vi "App - analyze RUS V6.vi"() -> ()   [LabVIEW 2015] (continued)
"Gamma"=0.06930828334440148, "phase"=3.842055847945363, "Q"=9613.327185902557, "Norm  Ampl"=0.033076114874311065, "z (inf)"=0.3276101846222711-0.3608645481780698i, "4corners"={"z (-pi/2)"=-0.3448645481780698-0.3036101846222711i, "z(inf)"=0.3276101846222711-0.3608645481780698i, "z (pi/2)"=0.3848645481780698+0.3116101846222711i, "z center"=0.020000000000000018+0.0040000000000000036i, "z(0)"=-0.28761018462227106+0.3688645481780698i, "radius"=0.4772317719940016}}, "timestamp(min)"=784.3500000014901, "timestamp"=timestamp(3493774882 s since 1904-01-01), "Magn Field(T)"=0.0}, {"temperature"=82.621, "lorentzian"={"Amplitude"=0.0006972416872469319, "omega(0)"=666.2547956648915, "Gamma"=0.06870985924393977, "phase"=3.8031954056849293, "Q"=9696.6403802327, "Norm  Ampl"=0.0324925976743957, "z (inf)"=0.2945387188362177-0.3771187551409229i, "4corners"={"z (-pi/2)"=-0.3691187551409229-0.2945387188362177i, "z(inf)"=0.2945387188362177-0.3771187551409229i, "z (pi/2)"=0.3771187551409229+0.2865387188362177i, "z center"=0.0040000000000000036-0.0040000000000000036i, "z(0)"=-0.2865387188362177+0.3691187551409229i, "radius"=0.4728957100470491}}, "timestamp(min)"=785.6666666641831, "timestamp"=timestamp(3493774961 s since 1904-01-01), "Magn Field(T)"=0.0}, {"temperature"=82.529, "lorentzian"={"Amplitude"=0.000685912737977901, "omega(0)"=666.2349515696993, "Gamma"=0.06796469782412583, "phase"=3.797698565029673, "Q"=9802.6618656311, "Norm  Ampl"=0.03238343021688376, "z (inf)"=0.29466641947231914-0.3735457173210897i, "4corners"={"z (-pi/2)"=-0.3735457173210897-0.28666641947231913i, "z(inf)"=0.29466641947231914-0.3735457173210897i, "z (pi/2)"=0.3815457173210897+0.29466641947231914i, "z center"=0.0040000000000000036+0.0040000000000000036i, "z(0)"=-0.28666641947231913+0.3815457173210897i, "radius"=0.47647427640571993}}, "timestamp(min)"=787.0, "timestamp"=timestamp(3493775041 s since 1904-01-01), "Magn Field(T)"=0.0}, {"temperature"=82.431, "lorentzian"={"Amplitude"=0.0006963027055650454, "omega(0)"=666.2143601194327, "Gamma"=0.06881606829798663, "phase"=3.7954467351945596, "Q"=9681.087231467485, "Norm  Ampl"=0.03280767739327282, "z (inf)"=0.3019798366954257-0.3744137256418556i, "4corners"={"z (-pi/2)"=-0.3664137256418556-0.2859798366954257i, "z(inf)"=0.3019798366954257-0.3744137256418556i, "z (pi/2)"=0.3904137256418556+0.2939798366954257i, "z center"=0.01200000000000001+0.0040000000000000036i, "z(0)"=-0.2779798366954257+0.3824137256418556i, "radius"=0.47674443200110406}}, "timestamp(min)"=788.3166666701436, "timestamp"=timestamp(3493775120 s since 1904-01-01), "Magn Field(T)"=0.0}, {"temperature"=82.336, "lorentzian"={"Amplitude"=0.0006854343320726252, "omega(0)"=666.1961380017648, "Gamma"=0.06908865385593883, "phase"=3.8305999287252495, "Q"=9642.627274094715, "Norm  Ampl"=0.03292832958384056, "z (inf)"=0.315014801293915-0.3638844014866976i, "4corners"={"z (-pi/2)"=-0.3558844014866976-0.299014801293915i, "z(inf)"=0.315014801293915-0.3638844014866976i, "z (pi/2)"=0.3798844014866976+0.307014801293915i, "z center"=0.01200000000000001+0.0040000000000000036i, "z(0)"=-0.291014801293915+0.3718844014866976i, "radius"=0.4766098012634827}}, "timestamp(min)"=789.6499999985099, "timestamp"=timestamp(3493775200 s since 1904-01-01), "Magn Field(T)"=0.0}, {"temperature"=82.244, "lorentzian"={"Amplitude"=0.0006602362683779066, "omega(0)"=666.1741792701555, "Gamma"=0.0652446126147674, "phase"=3.7900476591164622, "Q"=10210.408991214921, "Norm  Ampl"=0.030878877626074063, "z (inf)"=0.29783931461227364-0.373211480111581i, "4corners"={"z (-pi/2)"=-0.365211480111581-0.28183931461227363i, "z(inf)"=0.29783931461227364-0.373211480111581i, "z (pi/2)"=0.389211480111581+0.28983931461227364i, "z center"=0.01200000000000001+0.0040000000000000036i, "z(0)"=-0.2738393146122736+0.381211480111581i, "radius"=0.4732785802315419}}, "timestamp(min)"=790.9666666686535, "timestamp"=timestamp(3493775279 s since 1904-01-01), "Magn Field(T)"=0.0}, {"temperature"=82.149, "lorentzian"={"Amplitude"=0.0006811288853866493, "omega(0)"=666.1532060539795, "Gamma"=0.06653353924100215, "phase"=3.7827073809377345, "Q"=10012.291750195276, "Norm  Ampl"=0.031598979917904606, "z (inf)"=0.3040523510850292-0.37662541887555895i, "4corners"={"z (-pi/2)"=-0.36062541887555893-0.2800523510850292i, "z(inf)"=0.3040523510850292-0.37662541887555895i, "z (pi/2)"=0.40062541887555897+0.2880523510850292i, "z center"=0.020000000000000018+0.0040000000000000036i, "z(0)"=-0.26405235108502917+0.38462541887555896i, "radius"=0.47493309807922146}}, "timestamp(min)"=792.3000000044703, "timestamp"=timestamp(3493775359 s since 1904-01-01), "Magn Field(T)"=0.0}, {"temperature"=82.054, "lorentzian"={"Amplitude"=0.000661808176586954, "omega(0)"=666.134360050069, "Gamma"=0.06556456826571257, "phase"=3.7898177466936205, "Q"=10159.974780134844, "Norm  Ampl"=0.031199942872906523, "z (inf)"=0.30731473932842324-0.375339694559866i, "4corners"={"z (-pi/2)"=-0.359339694559866-0.2833147393284232i, "z(inf)"=0.30731473932842324-0.375339694559866i, "z (pi/2)"=0.399339694559866+0.2913147393284232i, "z center"=0.020000000000000018+0.0040000000000000036i, "z(0)"=-0.2673147393284232+0.383339694559866i, "radius"=0.475865908953491}}, "timestamp(min)"=793.6166666671634, "timestamp"=timestamp(3493775438 s since 1904-01-01), "Magn Field(T)"=0.0}, {"temperature"=81.963, "lorentzian"={"Amplitude"=0.0007965856787640092, "omega(0)"=666.1144609518154, "Gamma"=0.08199233511572589, "phase"=3.7672280161012996, "Q"=8124.106479119615, "Norm  Ampl"=0.037819800524082445, "z (inf)"=0.2901196948892255-0.3698934585888571i, "4corners"={"z (-pi/2)"=-0.35389345858885707-0.2661196948892255i, "z(inf)"=0.2901196948892255-0.3698934585888571i, "z (pi/2)"=0.3938934585888571+0.2741196948892255i, "z center"=0.020000000000000018+0.0040000000000000036i, "z(0)"=-0.2501196948892255+0.3778934585888571i, "radius"=0.4612601954890381}}, "timestamp(min)"=794.9500000029802, "timestamp"=timestamp(3493775518 s since 1904-01-01), "Magn Field(T)"=0.0}, {"temperature"=81.869, "lorentzian"={"Amplitude"=0.0006443086136346408, "omega(0)"=666.0941688470095, "Gamma"=0.06407247567602045, "phase"=3.7714167781112358, "Q"=10395.948678728824, "Norm  Ampl"=0.030440609010703657, "z (inf)"=0.29183309179237815-0.37994026371105843i, "4corners"={"z (-pi/2)"=-0.3719402637110584-0.27583309179237814i, "z(inf)"=0.29183309179237815-0.37994026371105843i, "z (pi/2)"=0.39594026371105845+0.28383309179237814i, "z center"=0.01200000000000001+0.0040000000000000036i, "z(0)"=-0.26783309179237813+0.38794026371105844i, "radius"=0.4750965011033007}}, "timestamp(min)"=796.2666666656733, "timestamp"=timestamp(3493775597 s since 1904-01-01), "Magn Field(T)"=0.0}, {"temperature"=81.779, "lorentzian"={"Amplitude"=0.0006410550959364764, "omega(0)"=666.0718120080683, "Gamma"=0.06459974834946221, "phase"=3.766353234357599, "Q"=10310.74932993316, "Norm  Ampl"=0.030568951865481662, "z (inf)"=0.2967793225918045-0.37981843110506236i, "4corners"={"z (-pi/2)"=-0.36381843110506235-0.2727793225918045i, "z(inf)"=0.2967793225918045-0.37981843110506236i, "z (pi/2)"=0.4038184311050624+0.2807793225918045i, "z center"=0.020000000000000018+0.0040000000000000036i, "z(0)"=-0.25677932259180447+0.38781843110506237i, "radius"=0.473205432629772}}, "timestamp(min)"=797.6000000014901, "timestamp"=timestamp(3493775677 s since 1904-01-01), "Magn Field(T)"=0.0}, {"temperature"=81.683, "lorentzian"={"Amplitude"=0.0006076266096898992, "omega(0)"=666.0514464195873, "Gamma"=0.06143889388749609, "phase"=3.7181106941402633, "Q"=10840.876263808203, "Norm  Ampl"=0.028912749616661376, "z (inf)"=0.27652437351805453-0.39852955831027087i, "4corners"={"z (-pi/2)"=-0.37452955831027085-0.2605243735180545i, "z(inf)"=0.27652437351805453-0.39852955831027087i, "z (pi/2)"=0.4145295583102709+0.2525243735180545i, "z center"=0.020000000000000018-0.0040000000000000036i, "z(0)"=-0.2365243735180545+0.39052955831027086i, "radius"=0.470593589617759}}, "timestamp(min)"=798.9166666641831, "timestamp"=timestamp(3493775756 s since 1904-01-01), "Magn Field(T)"=0.0}, {"temperature"=81.594, "lorentzian"={"Amplitude"=0.0006072936500237139, "omega(0)"=666.0325514837056, "Gamma"=0.06113714546082676, "phase"=3.728224240712266, "Q"=10894.07342235927, "Norm  Ampl"=0.028993515076990304, "z (inf)"=0.2745182904821208-0.3989495768812215i, "4corners"={"z (-pi/2)"=-0.3829495768812215-0.2665182904821208i, "z(inf)"=0.2745182904821208-0.3989495768812215i, "z (pi/2)"=0.4069495768812215+0.25851829048212077i, "z center"=0.01200000000000001-0.0040000000000000036i, "z(0)"=-0.25051829048212076+0.3909495768812215i, "radius"=0.47423730464432157}}, "timestamp(min)"=800.2333333343267, "timestamp"=timestamp(3493775835 s since 1904-01-01), "Magn Field(T)"=0.0}, {"temperature"=81.501, "lorentzian"={"Amplitude"=0.0005642204027786367, "omega(0)"=666.009795226544, "Gamma"=0.05680859204037456, "phase"=3.653534363936537, "Q"=11723.751131751385, "Norm  Ampl"=0.02670106809576054, "z (inf)"=0.250248223487721-0.4057594372375562i, "4corners"={"z (-pi/2)"=-0.3897594372375562-0.226248223487721i, "z(inf)"=0.250248223487721-0.4057594372375562i, "z (pi/2)"=0.4297594372375562+0.234248223487721i, "z center"=0.020000000000000018+0.0040000000000000036i, "z(0)"=-0.210248223487721+0.4137594372375562i, "radius"=0.4700181281870841}}, "timestamp(min)"=801.5666666701436, "timestamp"=timestamp(3493775915 s since 1904-01-01), "Magn Field(T)"=0.0}, {"temperature"=81.408, "lorentzian"={"Amplitude"=0.0007103334002699531, "omega(0)"=665.9953474434808, "Gamma"=0.07133253713577505, "phase"=3.83036810247925, "Q"=9336.487585964014, "Norm  Ampl"=0.033760580923824425, "z (inf)"=0.3128159431546857-0.36938738782429087i, "4corners"={"z (-pi/2)"=-0.35338738782429086-0.3048159431546857i, "z(inf)"=0.3128159431546857-0.36938738782429087i, "z (pi/2)"=0.3773873878242909+0.2968159431546857i, "z center"=0.01200000000000001-0.0040000000000000036i, "z(0)"=-0.2888159431546857+0.36138738782429086i, "radius"=0.4732844544638054}}, "timestamp(min)"=802.8833333328366, "timestamp"=timestamp(3493775994 s since 1904-01-01), "Magn Field(T)"=0.0}, {"temperature"=81.32, "lorentzian"={"Amplitude"=0.000582609698476251, "omega(0)"=665.9751947106768, "Gamma"=0.05812976574150381, "phase"=3.7119036338106897, "Q"=11456.698409420565, "Norm  Ampl"=0.027685811339377663, "z (inf)"=0.2771384682011788-0.4048972692221223i, "4corners"={"z (-pi/2)"=-0.3808972692221223-0.2611384682011788i, "z(inf)"=0.2771384682011788-0.4048972692221223i, "z (pi/2)"=0.42089726922212234+0.2531384682011788i, "z center"=0.020000000000000018-0.0040000000000000036i, "z(0)"=-0.2371384682011788+0.3968972692221223i, "radius"=0.47627598333172694}}, "timestamp(min)"=804.2000000029802, "timestamp"=timestamp(3493776073 s since 1904-01-01), "Magn Field(T)"=0.0}, {"temperature"=81.229, "lorentzian"={"Amplitude"=0.0006264615993985428, "omega(0)"=665.9553477881376, "Gamma"=0.06192296967531283, "phase"=3.747605050615115, "Q"=10754.57703789096, "Norm  Ampl"=0.02952636058821417, "z (inf)"=0.29959634287061726-0.395914010914744i, "4corners"={"z (-pi/2)"=-0.36391401091474396-0.27559634287061724i, "z(inf)"=0.29959634287061726-0.395914010914744i, "z (pi/2)"=0.419914010914744+0.26759634287061723i, "z center"=0.028000000000000025-0.0040000000000000036i, "z(0)"=-0.2435963428706172+0.387914010914744i, "radius"=0.4768240403041524}}, "timestamp(min)"=805.5333333313465, "timestamp"=timestamp(3493776153 s since 1904-01-01), "Magn Field(T)"=0.0}, {"temperature"=81.134, "lorentzian"={"Amplitude"=0.0005982305706101968, "omega(0)"=665.9343195300057, "Gamma"=0.060064378770215206, "phase"=3.6726072791552684, "Q"=11087.009191881129, "Norm  Ampl"=0.028368216383599845, "z (inf)"=0.25917513837394046-0.41125859074294846i, "4corners"={"z (-pi/2)"=-0.38725859074294844-0.24317513837394047i, "z(inf)"=0.25917513837394046-0.41125859074294846i, "z (pi/2)"=0.4272585907429485+0.23517513837394047i, "z center"=0.020000000000000018-0.0040000000000000036i, "z(0)"=-0.21917513837394045+0.40325859074294845i, "radius"=0.4722968415627252}}, "timestamp(min)"=806.8500000014901, "timestamp"=timestamp(3493776232 s since 1904-01-01), "Magn Field(T)"=0.0}, {"temperature"=81.047, "lorentzian"={"Amplitude"=0.0005436604150965886, "omega(0)"=665.9126957276022, "Gamma"=0.054391615502220096, "phase"=3.623436848836922, "Q"=12242.929164338238, "Norm  Ampl"=0.025547222809101933, "z (inf)"=0.23766121910248528-0.4122123499501512i, "4corners"={"z (-pi/2)"=-0.3962123499501512-0.21366121910248526i, "z(inf)"=0.23766121910248528-0.4122123499501512i, "z (pi/2)"=0.43621234995015123+0.22166121910248526i, "z center"=0.020000000000000018+0.0040000000000000036i, "z(0)"=-0.19766121910248524+0.4202123499501512i, "radius"=0.4696904582298934}}, "timestamp(min)"=808.183333337307, "timestamp"=timestamp(3493776312 s since 1904-01-01), "Magn Field(T)"=0.0}, {"temperature"=80.958, "lorentzian"={"Amplitude"=0.0005359009844102671, "omega(0)"=665.893856538965, "Gamma"=0.05365668737469352, "phase"=3.6524069233354184, "Q"=12410.267743308827, "Norm  Ampl"=0.025203485884419292, "z (inf)"=0.24163913197447767-0.405756529475521i, "4corners"={"z (-pi/2)"=-0.397756529475521-0.22563913197447766i, "z(inf)"=0.24163913197447767-0.405756529475521i, "z (pi/2)"=0.421756529475521+0.23363913197447767i, "z center"=0.01200000000000001+0.0040000000000000036i, "z(0)"=-0.21763913197447765+0.413756529475521i, "radius"=0.46971751551524565}}, "timestamp(min)"=809.5, "timestamp"=timestamp(3493776391 s since 1904-01-01), "Magn Field(T)"=0.0}, {"temperature"=80.871, "lorentzian"={"Amplitude"=0.0005271309388079498, "omega(0)"=665.8735587517352, "Gamma"=0.0529251400813889, "phase"=3.6114149158792337, "Q"=12581.422698697577, "Norm  Ampl"=0.025135729535680076, "z (inf)"=0.23501395823116833-0.41947062787261763i, "4corners"={"z (-pi/2)"=-0.4034706278726176-0.2110139582311683i, "z(inf)"=0.23501395823116833-0.41947062787261763i, "z (pi/2)"=0.44347062787261765+0.21901395823116832i, "z center"=0.020000000000000018+0.0040000000000000036i, "z(0)"=-0.1950139582311683+0.42747062787261764i, "radius"=0.47492986314303676}}, "timestamp(min)"=810.8166666701436, "timestamp"=timestamp(3493776470 s since 1904-01-01), "Magn Field(T)"=0.0}, {"temperature"=80.778, "lorentzian"={"Amplitude"=0.0005267654786186403, "omega(0)"=665.8525097864081, "Gamma"=0.052338348231804756, "phase"=3.5786985819989203, "Q"=12722.077258483016, "Norm  Ampl"=0.024789112532138686, "z (inf)"=0.22049751946201726-0.4331013206689819i, "4corners"={"z (-pi/2)"=-0.40910132066898186-0.20449751946201725i, "z(inf)"=0.22049751946201726-0.4331013206689819i, "z (pi/2)"=0.4491013206689819+0.19649751946201724i, "z center"=0.020000000000000018-0.0040000000000000036i, "z(0)"=-0.18049751946201723+0.4251013206689819i, "radius"=0.47363192323816855}}, "timestamp(min)"=812.1499999985099, "timestamp"=timestamp(3493776550 s since 1904-01-01), "Magn Field(T)"=0.0}, {"temperature"=80.688, "lorentzian"={"Amplitude"=0.0005087274085603998, "omega(0)"=665.8348091435408, "Gamma"=0.05138178107814259, "phase"=3.594454792183561, "Q"=12958.577829969032, "Norm  Ampl"=0.024069545346628345, "z (inf)"=0.22496393075941817-0.42522515487487184i, "4corners"={"z (-pi/2)"=-0.4012251548748718-0.20896393075941816i, "z(inf)"=0.22496393075941817-0.42522515487487184i, "z (pi/2)"=0.44122515487487185+0.20096393075941815i, "z center"=0.020000000000000018-0.0040000000000000036i, "z(0)"=-0.18496393075941814+0.41722515487487183i, "radius"=0.46844513447330344}}, "timestamp(min)"=813.4666666686535, "timestamp"=timestamp(3493776629 s since 1904-01-01), "Magn Field(T)"=0.0}, {"temperature"=80.602, "lorentzian"={"Amplitude"=0.0004882899356981653, "omega(0)"=665.8124994707074, "Gamma"=0.04910380713640485, "phase"=3.547437034982565, "Q"=13559.284672594838, "Norm  Ampl"=0.023246840914470077, "z (inf)"=0.20690464043593387-0.4389659744864196i, "4corners"={"z (-pi/2)"=-0.4149659744864196-0.19090464043593386i, "z(inf)"=0.20690464043593387-0.4389659744864196i, "z (pi/2)"=0.4549659744864196+0.18290464043593385i, "z center"=0.020000000000000018-0.0040000000000000036i, "z(0)"=-0.16690464043593384+0.4309659744864196i, "radius"=0.4734223733384454}}, "timestamp(min)"=814.8000000044703, "timestamp"=timestamp(3493776709 s since 1904-01-01), "Magn Field(T)"=0.0}, {"temperature"=80.512, "lorentzian"={"Amplitude"=0.0004667929339879065, "omega(0)"=665.7921823307441, "Gamma"=0.046744260040372576, "phase"=3.511637879553154, "Q"=14243.292796927488, "Norm  Ampl"=0.022223516509620588, "z (inf)"=0.19194204316769328-0.4472464791600908i, "4corners"={"z (-pi/2)"=-0.4232464791600908-0.17594204316769327i, "z(inf)"=0.19194204316769328-0.4472464791600908i, "z (pi/2)"=0.4632464791600908+0.16794204316769326i, "z center"=0.020000000000000018-0.0040000000000000036i, "z(0)"=-0.15194204316769325+0.4392464791600908i, "radius"=0.4754277100637885}}, "timestamp(min)"=816.1166666671634, "timestamp"=timestamp(3493776788 s since 1904-01-01), "Magn Field(T)"=0.0}, {"temperature"=80.428, "lorentzian"={"Amplitude"=0.0004489209270346126, "omega(0)"=665.770336097026, "Gamma"=0.044967586490377534, "phase"=3.4772880687633405, "Q"=14805.560806326395, "Norm  Ampl"=0.021387258385219494, "z (inf)"=0.1766798725688283-0.45306685491684434i, "4corners"={"z (-pi/2)"=-0.4290668549168443-0.1606798725688283i, "z(inf)"=0.1766798725688283-0.45306685491684434i, "z (pi/2)"=0.46906685491684436+0.15267987256882828i, "z center"=0.020000000000000018-0.0040000000000000036i, "z(0)"=-0.13667987256882827+0.44506685491684433i, "radius"=0.475614994142416}}, "timestamp(min)"=817.433333337307, "timestamp"=timestamp(3493776867 s since 1904-01-01), "Magn Field(T)"=0.0}, {"temperature"=80.338, "lorentzian"={"Amplitude"=0.00044807774453631103, "omega(0)"=665.751169981811, "Gamma"=0.044783012994154305, "phase"=3.478549048664672, "Q"=14866.154049722247, "Norm  Ampl"=0.021488852823685116, "z (inf)"=0.17864413626604192-0.45685996368629533i, "4corners"={"z (-pi/2)"=-0.4328599636862953-0.1626441362660419i, "z(inf)"=0.17864413626604192-0.45685996368629533i, "z (pi/2)"=0.47285996368629535+0.1546441362660419i, "z center"=0.020000000000000018-0.0040000000000000036i, "z(0)"=-0.13864413626604188+0.4488599636862953i, "radius"=0.4798438378072091}}, "timestamp(min)"=818.7666666656733, "timestamp"=timestamp(3493776947 s since 1904-01-01), "Magn Field(T)"=0.0}, {"temperature"=80.249, "lorentzian"={"Amplitude"=0.0004339429327407474, "omega(0)"=665.7310500779857, "Gamma"=0.042797667772295565, "phase"=3.467881219083677, "Q"=15555.311416033208, "Norm  Ampl"=0.02057222058744532, "z (inf)"=0.17407396257240368-0.45932385686764793i, "4corners"={"z (-pi/2)"=-0.4353238568676479-0.15807396257240366i, "z(inf)"=0.17407396257240368-0.45932385686764793i, "z (pi/2)"=0.47532385686764794+0.15007396257240366i, "z center"=0.020000000000000018-0.0040000000000000036i, "z(0)"=-0.13407396257240364+0.4513238568676479i, "radius"=0.48068555270113206}}, "timestamp(min)"=820.0833333358169, "timestamp"=timestamp(3493777026 s since 1904-01-01), "Magn Field(T)"=0.0}, {"temperature"=80.163, "lorentzian"={"Amplitude"=0.0004318053404680994, "omega(0)"=665.7095388817693, "Gamma"=0.04251465906133632, "phase"=3.4410157944541444, "Q"=15658.352991172846, "Norm  Ampl"=0.020516700930109627, "z (inf)"=0.1623460091556352-0.4651079510202824i, "4corners"={"z (-pi/2)"=-0.4411079510202824-0.1463460091556352i, "z(inf)"=0.1623460091556352-0.4651079510202824i, "z (pi/2)"=0.4811079510202824+0.1383460091556352i, "z center"=0.020000000000000018-0.0040000000000000036i, "z(0)"=-0.12234600915563518+0.4571079510202824i, "radius"=0.4825794533718353}}, "timestamp(min)"=821.3999999985099, "timestamp"=timestamp(3493777105 s since 1904-01-01), "Magn Field(T)"=0.0}, {"temperature"=80.075, "lorentzian"={"Amplitude"=0.0004410954482919087, "omega(0)"=665.6890167901994, "Gamma"=0.043283815856253634, "phase"=3.455890711993292, "Q"=15379.628704663312, "Norm  Ampl"=0.021014667550651542, "z (inf)"=0.16209451338682376-0.46572534970148993i, "4corners"={"z (-pi/2)"=-0.4497253497014899-0.15409451338682376i, "z(inf)"=0.16209451338682376-0.46572534970148993i, "z (pi/2)"=0.47372534970148994+0.14609451338682375i, "z center"=0.01200000000000001-0.0040000000000000036i, "z(0)"=-0.13809451338682374+0.4577253497014899i, "radius"=0.4855086626475274}}, "timestamp(min)"=822.7333333343267, "timestamp"=timestamp(3493777185 s since 1904-01-01), "Magn Field(T)"=0.0}, {"temperature"=79.991, "lorentzian"={"Amplitude"=0.00045081873601942116, "omega(0)"=665.666392459161, "Gamma"=0.04417730101978429, "phase"=3.41518632314404, "Q"=15068.06384937482, "Norm  Ampl"=0.021340141879038124, "z (inf)"=0.1425186302592478-0.46908996594687835i, "4corners"={"z (-pi/2)"=-0.45308996594687834-0.1345186302592478i, "z(inf)"=0.1425186302592478-0.46908996594687835i, "z (pi/2)"=0.47708996594687836+0.12651863025924778i, "z center"=0.01200000000000001-0.0040000000000000036i, "z(0)"=-0.11851863025924778+0.46108996594687834i, "radius"=0.48305671434027153}}, "timestamp(min)"=824.0500000044703, "timestamp"=timestamp(3493777264 s since 1904-01-01), "Magn Field(T)"=0.0}, {"temperature"=79.903, "lorentzian"={"Amplitude"=0.00041982693484479076, "omega(0)"=665.6483705534005, "Gamma"=0.04131522725547794, "phase"=3.4489219493632968, "Q"=16111.453688425323, "Norm  Ampl"=0.019830531774632107, "z (inf)"=0.15720110058856143-0.461491616562412i, "4corners"={"z (-pi/2)"=-0.445491616562412-0.14920110058856142i, "z(inf)"=0.15720110058856143-0.461491616562412i, "z (pi/2)"=0.469491616562412+0.14120110058856142i, "z center"=0.01200000000000001-0.0040000000000000036i, "z(0)"=-0.1332011005885614+0.453491616562412i, "radius"=0.4799811859198426}}, "timestamp(min)"=825.3833333328366, "timestamp"=timestamp(3493777344 s since 1904-01-01), "Magn Field(T)"=0.0}, {"temperature"=79.817, "lorentzian"={"Amplitude"=0.0004473207739177375, "omega(0)"=665.6281709996543, "Gamma"=0.04424370195385826, "phase"=3.458741913142453, "Q"=15044.585819103422, "Norm  Ampl"=0.021108986152116926, "z (inf)"=0.1607902810627609-0.4573130004493936i, "4corners"={"z (-pi/2)"=-0.4413130004493936-0.15279028106276088i, "z(inf)"=0.1607902810627609-0.4573130004493936i, "z (pi/2)"=0.4653130004493936+0.14479028106276087i, "z center"=0.01200000000000001-0.0040000000000000036i, "z(0)"=-0.13679028106276087+0.4493130004493936i, "radius"=0.47710714112782604}}, "timestamp(min)"=826.7000000029802, "timestamp"=timestamp(3493777423 s since 1904-01-01), "Magn Field(T)"=0.0}, {"temperature"=79.734, "lorentzian"={"Amplitude"=0.0004310190190592046, "omega(0)"=665.6073287703097, "Gamma"=0.04260556553164946, "phase"=3.3897140798024243, "Q"=15622.544155079097, "Norm  Ampl"=0.020208251339171045, "z (inf)"=0.13648267088154692-0.46378460946108147i, "4corners"={"z (-pi/2)"=-0.43978460946108144-0.12048267088154692i, "z(inf)"=0.13648267088154692-0.46378460946108147i, "z (pi/2)"=0.4797846094610815+0.11248267088154691i, "z center"=0.020000000000000018-0.0040000000000000036i, "z(0)"=-0.0964826708815469+0.45578460946108146i, "radius"=0.47431013030819613}}, "timestamp(min)"=828.0166666656733, "timestamp"=timestamp(3493777502 s since 1904-01-01), "Magn Field(T)"=0.0}, {"temperature"=79.645, "lorentzian"={"Amplitude"=0.0004937499674397325, "omega(0)"=665.5905919172243, "Gamma"=0.04842744547368939, "phase"=3.596201043814433, "Q"=13744.078082310563, "Norm  Ampl"=0.02365453214362621, "z (inf)"=0.2264848572256194-0.43484234277978495i, "4corners"={"z (-pi/2)"=-0.42684234277978494-0.21048485722561938i, "z(inf)"=0.2264848572256194-0.43484234277978495i, "z (pi/2)"=0.45084234277978497+0.2184848572256194i, "z center"=0.01200000000000001+0.0040000000000000036i, "z(0)"=-0.20248485722561937+0.44284234277978496i, "radius"=0.48845302312048866}}, "timestamp(min)"=829.3500000014901, "timestamp"=timestamp(3493777582 s since 1904-01-01), "Magn Field(T)"=0.0}, {"temperature"=79.564, "lorentzian"={"Amplitude"=0.00040885006198574856, "omega(0)"=665.5700736081353, "Gamma"=0.04004258239584053, "phase"=3.476858345479039, "Q"=16621.557197002167, "Norm  Ampl"=0.019088365277797854, "z (inf)"=0.17684441669665446-0.4541603007110035i, "4corners"={"z (-pi/2)"=-0.4301603007110035-0.16084441669665445i, "z(inf)"=0.17684441669665446-0.4541603007110035i, "z (pi/2)"=0.4701603007110035+0.15284441669665444i, "z center"=0.020000000000000018-0.0040000000000000036i, "z(0)"=-0.13684441669665443+0.4461603007110035i, "radius"=0.47670165448122254}}, "timestamp(min)"=830.6666666641831, "timestamp"=timestamp(3493777661 s since 1904-01-01), "Magn Field(T)"=0.0}, {"temperature"=79.476, "lorentzian"={"Amplitude"=0.00042495979141987184, "omega(0)"=665.5494957126687, "Gamma"=0.04195737945665875, "phase"=3.493368033553565, "Q"=15862.51344415277, "Norm  Ampl"=0.01992681463808725, "z (inf)"=0.1836442305829716-0.44984637431067337i, "4corners"={"z (-pi/2)"=-0.42584637431067335-0.1676442305829716i, "z(inf)"=0.1836442305829716-0.44984637431067337i, "z (pi/2)"=0.4658463743106734+0.15964423058297159i, "z center"=0.020000000000000018-0.0040000000000000036i, "z(0)"=-0.14364423058297157+0.44184637431067336i, "radius"=0.4749299145021988}}, "timestamp(min)"=831.9833333343267, "timestamp"=timestamp(3493777740 s since 1904-01-01), "Magn Field(T)"=0.0}, {"temperature"=79.39, "lorentzian"={"Amplitude"=0.00038786955968295433, "omega(0)"=665.5288680893714, "Gamma"=0.03759056507164493, "phase"=3.4134184071386273, "Q"=17704.678469741568, "Norm  Ampl"=0.01789292667738704, "z (inf)"=0.1478002232066598-0.46251770545494364i, "4corners"={"z (-pi/2)"=-0.4385177054549436-0.1318002232066598i, "z(inf)"=0.1478002232066598-0.46251770545494364i, "z (pi/2)"=0.47851770545494365+0.12380022320665979i, "z center"=0.020000000000000018-0.0040000000000000036i, "z(0)"=-0.10780022320665977+0.45451770545494363i, "radius"=0.475995150466198}}, "timestamp(min)"=833.3166666701436, "timestamp"=timestamp(3493777820 s since 1904-01-01), "Magn Field(T)"=0.0}, {"temperature"=79.307, "lorentzian"={"Amplitude"=0.00039486048335689604, "omega(0)"=665.5099899305785, "Gamma"=0.03858281710445579, "phase"=3.4091675266271304, "Q"=17248.869830547475, "Norm  Ampl"=0.01824836061418064, "z (inf)"=0.14504908265784147-0.46013546518605314i, "4corners"={"z (-pi/2)"=-0.4361354651860531-0.12904908265784146i, "z(inf)"=0.14504908265784147-0.46013546518605314i, "z (pi/2)"=0.47613546518605315+0.12104908265784145i, "z center"=0.020000000000000018-0.0040000000000000036i, "z(0)"=-0.10504908265784144+0.45213546518605313i, "radius"=0.4729659984333597}}, "timestamp(min)"=834.6333333328366, "timestamp"=timestamp(3493777899 s since 1904-01-01), "Magn Field(T)"=0.0}, {"temperature"=79.224, "lorentzian"={"Amplitude"=0.0003845370054352556, "omega(0)"=665.4902430620257, "Gamma"=0.03743783061492319, "phase"=3.4010110518499768, "Q"=17775.876222826675, "Norm  Ampl"=0.01788160860855218, "z (inf)"=0.1345221260483211-0.465652766112582i, "4corners"={"z (-pi/2)"=-0.449652766112582-0.12652212604832108i, "z(inf)"=0.1345221260483211-0.465652766112582i, "z (pi/2)"=0.473652766112582+0.11852212604832109i, "z center"=0.01200000000000001-0.0040000000000000036i, "z(0)"=-0.11052212604832108+0.457652766112582i, "radius"=0.4776347431152795}}, "timestamp(min)"=835.9666666686535, "timestamp"=timestamp(3493777979 s since 1904-01-01), "Magn Field(T)"=0.0}, {"temperature"=79.141, "lorentzian"={"Amplitude"=0.0003670811848988743, "omega(0)"=665.4692472952553, "Gamma"=0.035318217866197155, "phase"=3.3464602427490036, "Q"=18842.09587857409, "Norm  Ampl"=0.016835680164561606, "z (inf)"=0.10897570331399178-0.47071695928266144i, "4corners"={"z (-pi/2)"=-0.4547169592826614-0.10097570331399178i, "z(inf)"=0.10897570331399178-0.47071695928266144i, "z (pi/2)"=0.47871695928266145+0.09297570331399177i, "z center"=0.01200000000000001-0.0040000000000000036i, "z(0)"=-0.08497570331399176+0.46271695928266143i, "radius"=0.47668543832940485}}, "timestamp(min)"=837.2833333313465, "timestamp"=timestamp(3493778058 s since 1904-01-01), "Magn Field(T)"=0.0}, {"temperature"=79.055, "lorentzian"={"Amplitude"=0.0003630000157983062, "omega(0)"=665.4499677322567, "Gamma"=0.03492637330483988, "phase"=3.3445475874819053, "Q"=19052.9363562647, "Norm  Ampl"=0.016732964798190038, "z (inf)"=0.10856804346537254-0.4732592802307583i, "4corners"={"z (-pi/2)"=-0.4572592802307583-0.10056804346537253i, "z(inf)"=0.10856804346537254-0.4732592802307583i, "z (pi/2)"=0.4812592802307583+0.09256804346537252i, "z center"=0.01200000000000001-0.0040000000000000036i, "z(0)"=-0.08456804346537251+0.4652592802307583i, "radius"=0.47909253709635197}}, "timestamp(min)"=838.6000000014901, "timestamp"=timestamp(3493778137 s since 1904-01-01), "Magn Field(T)"=0.0}, {"temperature"=78.972, "lorentzian"={"Amplitude"=0.00035124627344787984, "omega(0)"=665.4301516983661, "Gamma"=0.03353544809665225, "phase"=3.328046862744741, "Q"=19842.590138665662, "Norm  Ampl"=0.016004873562181932, "z (inf)"=0.1004710162912438-0.47298053908915594i, "4corners"={"z (-pi/2)"=-0.4569805390891559-0.0924710162912438i, "z(inf)"=0.1004710162912438-0.47298053908915594i, "z (pi/2)"=0.48098053908915595+0.08447101629124379i, "z center"=0.01200000000000001-0.0040000000000000036i, "z(0)"=-0.07647101629124378+0.46498053908915593i, "radius"=0.47725241410385855}}, "timestamp(min)"=839.933333337307, "timestamp"=timestamp(3493778217 s since 1904-01-01), "Magn Field(T)"=0.0}, {"temperature"=78.889, "lorentzian"={"Amplitude"=0.0008301116528174503, "omega(0)"=0.0, "Gamma"=0.0, "phase"=4.0108774417714885, "Q"=5965.026272969477, "Norm  Ampl"=0.03891514556991122, "z (inf)"=0.3585098440365777-0.3731676578774482i, "4corners"={"z (-pi/2)"=-0.1331676578774482-0.41450984403657776i, "z(inf)"=0.3585098440365777-0.3731676578774482i, "z (pi/2)"=0.31716765787744816+0.11850984403657772i, "z center"=0.09199999999999997-0.14800000000000002i, "z(0)"=-0.17450984403657777+0.07716765787744814i, "radius"=0.3488953584134024}}, "timestamp(min)"=841.25, "timestamp"=timestamp(3493778296 s since 1904-01-01), "Magn Field(T)"=0.0}, {"temperature"=78.806, "lorentzian"={"Amplitude"=0.0007610200428348603, "omega(0)"=0.0, "Gamma"=0.0, "phase"=3.8882769320564767, "Q"=8601.366182630625, "Norm  Ampl"=0.03098927927002168, "z (inf)"=0.25210338177196456-0.39403162340529885i, "4corners"={"z (-pi/2)"=-0.3140316234052989-0.37210338177196456i, "z(inf)"=0.25210338177196456-0.39403162340529885i, "z (pi/2)"=0.27403162340529885+0.1721033817719646i, "z center"=-0.020000000000000018-0.09999999999999998i, "z(0)"=-0.2921033817719646+0.1940316234052989i, "radius"=0.40061807988918197}}, "timestamp(min)"=842.5666666701436, "timestamp"=timestamp(3493778375 s since 1904-01-01), "Magn Field(T)"=0.0}, {"temperature"=78.721, "lorentzian"={"Amplitude"=0.00031162361885979584, "omega(0)"=0.0, "Gamma"=0.0, "phase"=3.304961535631265, "Q"=20803.26616116804, "Norm  Ampl"=0.013030724756859974, "z (inf)"=-0.009731683131084592-0.40602093996801597i, "4corners"={"z (-pi/2)"=-0.478020939968016-0.07026831686891542i, "z(inf)"=-0.009731683131084592-0.40602093996801597i, "z (pi/2)"=0.32602093996801595+0.062268316868915416i, "z center"=-0.07600000000000001-0.0040000000000000036i, "z(0)"=-0.14226831686891545+0.39802093996801596i, "radius"=0.40744610194896463}}, "timestamp(min)"=843.8999999985099, "timestamp"=timestamp(3493778455 s since 1904-01-01), "Magn Field(T)"=0.0}, {"temperature"=78.641, "lorentzian"={"Amplitude"=0.0003469733840605032, "omega(0)"=665.3000947405819, "Gamma"=0.03666623179697319, "phase"=3.4559757315265314, "Q"=18144.763236769333, "Norm  Ampl"=0.017226418900473012, "z (inf)"=0.18128143706592992-0.4507900114857177i, "4corners"={"z (-pi/2)"=-0.41079001148571764-0.1492814370659299i, "z(inf)"=0.18128143706592992-0.4507900114857177i, "z (pi/2)"=0.4827900114857177+0.14128143706592988i, "z center"=0.03600000000000003-0.0040000000000000036i, "z(0)"=-0.10928143706592985+0.44279001148571767i, "radius"=0.46981699662671794}}, "timestamp(min)"=845.2166666686535, "timestamp"=timestamp(3493778534 s since 1904-01-01), "Magn Field(T)"=0.0}, {"temperature"=78.559, "lorentzian"={"Amplitude"=0.0002633710378356322, "omega(0)"=665.2801278621953, "Gamma"=0.028182977879510615, "phase"=3.4382041539112964, "Q"=23605.74282485111, "Norm  Ampl"=0.013078354485010291, "z (inf)"=0.15563361676688114-0.44778751707019715i, "4corners"={"z (-pi/2)"=-0.42378751707019713-0.13963361676688113i, "z(inf)"=0.15563361676688114-0.44778751707019715i, "z (pi/2)"=0.46378751707019716+0.13163361676688112i, "z center"=0.020000000000000018-0.0040000000000000036i, "z(0)"=-0.11563361676688111+0.43978751707019714i, "radius"=0.46405154703394286}}, "timestamp(min)"=846.5500000044703, "timestamp"=timestamp(3493778614 s since 1904-01-01), "Magn Field(T)"=0.0}, {"temperature"=78.479, "lorentzian"={"Amplitude"=0.00026741351353309494, "omega(0)"=665.2619142461758, "Gamma"=0.02872568487925299, "phase"=3.5885166425038406, "Q"=23159.131524368233, "Norm  Ampl"=0.013282283181435752, "z (inf)"=0.21983924059518142-0.4129685767860478i, "4corners"={"z (-pi/2)"=-0.3969685767860478-0.1958392405951814i, "z(inf)"=0.21983924059518142-0.4129685767860478i, "z (pi/2)"=0.43696857678604784+0.2038392405951814i, "z center"=0.020000000000000018+0.0040000000000000036i, "z(0)"=-0.1798392405951814+0.4209685767860478i, "radius"=0.4623835162596533}}, "timestamp(min)"=847.8666666671634, "timestamp"=timestamp(3493778693 s since 1904-01-01), "Magn Field(T)"=0.0}, {"temperature"=78.395, "lorentzian"={"Amplitude"=0.0002736558669474432, "omega(0)"=665.2441266774955, "Gamma"=0.02923413654907257, "phase"=3.706685269521818, "Q"=22755.730293617988, "Norm  Ampl"=0.01360923632841206, "z (inf)"=0.2692861342823963-0.38915445282846434i, "4corners"={"z (-pi/2)"=-0.3731544528284643-0.24528613428239626i, "z(inf)"=0.2692861342823963-0.38915445282846434i, "z (pi/2)"=0.41315445282846436+0.25328613428239627i, "z center"=0.020000000000000018+0.0040000000000000036i, "z(0)"=-0.22928613428239625+0.39715445282846434i, "radius"=0.46552551006825615}}, "timestamp(min)"=849.183333337307, "timestamp"=timestamp(3493778772 s since 1904-01-01), "Magn Field(T)"=0.0}, {"temperature"=78.313, "lorentzian"={"Amplitude"=0.0002701026151051536, "omega(0)"=665.2240080628333, "Gamma"=0.029121998975374923, "phase"=3.687779261469825, "Q"=22842.66298564654, "Norm  Ampl"=0.013530076904295783, "z (inf)"=0.2613282370238335-0.3930059447167146i, "4corners"={"z (-pi/2)"=-0.37700594471671456-0.2373282370238335i, "z(inf)"=0.2613282370238335-0.3930059447167146i, "z (pi/2)"=0.4170059447167146+0.2453282370238335i, "z center"=0.020000000000000018+0.0040000000000000036i, "z(0)"=-0.22132823702383347+0.4010059447167146i, "radius"=0.4645998688392438}}, "timestamp(min)"=850.5166666656733, "timestamp"=timestamp(3493778852 s since 1904-01-01), "Magn Field(T)"=0.0}, {"temperature"=78.233, "lorentzian"={"Amplitude"=0.00019778742884725761, "omega(0)"=665.2045077919724, "Gamma"=0.021371395220282488, "phase"=3.5670951697593205, "Q"=31125.92794880613, "Norm  Ampl"=0.009948064688774712, "z (inf)"=0.20414223447958435-0.4199783970147834i, "4corners"={"z (-pi/2)"=-0.4119783970147834-0.18814223447958434i, "z(inf)"=0.20414223447958435-0.4199783970147834i, "z (pi/2)"=0.4359783970147834+0.19614223447958434i, "z center"=0.01200000000000001+0.0040000000000000036i, "z(0)"=-0.18014223447958433+0.4279783970147834i, "radius"=0.4654850367155027}}, "timestamp(min)"=851.8333333358169, "timestamp"=timestamp(3493778931 s since 1904-01-01), "Magn Field(T)"=0.0}, {"temperature"=78.151, "lorentzian"={"Amplitude"=0.00017564595267696503, "omega(0)"=665.183555272565, "Gamma"=0.019189976087277332, "phase"=3.2201158903387377, "Q"=34663.07369260203, "Norm  Ampl"=0.008694611032951266, "z (inf)"=0.03954082649388515-0.4476847607482463i, "4corners"={"z (-pi/2)"=-0.4476847607482463-0.03154082649388514i, "z(inf)"=0.03954082649388515-0.4476847607482463i, "z (pi/2)"=0.4556847607482463+0.03954082649388515i, "z center"=0.0040000000000000036+0.0040000000000000036i, "z(0)"=-0.03154082649388514+0.4556847607482463i, "radius"=0.4530808685434301}}, "timestamp(min)"=853.1666666641831, "timestamp"=timestamp(3493779011 s since 1904-01-01), "Magn Field(T)"=0.0}, {"temperature"=78.071, "lorentzian"={"Amplitude"=0.00019961568008146176, "omega(0)"=665.170171669107, "Gamma"=0.02190790980665959, "phase"=3.2007471946877457, "Q"=30362.101064835857, "Norm  Ampl"=0.00880139115714775, "z (inf)"=-0.05224882205137665-0.39704220566019993i, "4corners"={"z (-pi/2)"=-0.47704220566019995-0.01975117794862335i, "z(inf)"=-0.05224882205137665-0.39704220566019993i, "z (pi/2)"=0.3250422056601999+0.02775117794862336i, "z center"=-0.07600000000000001+0.0040000000000000036i, "z(0)"=-0.09975117794862337+0.40504220566019994i, "radius"=0.40174490559899484}}, "timestamp(min)"=854.4833333343267, "timestamp"=timestamp(3493779090 s since 1904-01-01), "Magn Field(T)"=0.0}, {"temperature"=77.989, "lorentzian"={"Amplitude"=0.00033034126926953923, "omega(0)"=665.1523314137073, "Gamma"=0.03562891996885951, "phase"=3.3234983284640904, "Q"=18668.888419718187, "Norm  Ampl"=0.011390348763886537, "z (inf)"=-0.09816605010122248-0.3184191960869025i, "4corners"={"z (-pi/2)"=-0.4704191960869025-0.06183394989877756i, "z(inf)"=-0.09816605010122248-0.3184191960869025i, "z (pi/2)"=0.15841919608690247+0.05383394989877755i, "z center"=-0.15600000000000003-0.0040000000000000036i, "z(0)"=-0.21383394989877758+0.3104191960869025i, "radius"=0.3196939108410236}}, "timestamp(min)"=855.8000000044703, "timestamp"=timestamp(3493779169 s since 1904-01-01), "Magn Field(T)"=0.0}, {"temperature"=77.909, "lorentzian"={"Amplitude"=0.0002506126859092132, "omega(0)"=665.1325777519697, "Gamma"=0.027515735254439094, "phase"=3.261185853283691, "Q"=24172.80772625054, "Norm  Ampl"=0.013007065400587844, "z (inf)"=0.06039868023632579-0.47333723920034887i, "4corners"={"z (-pi/2)"=-0.46533723920034886-0.06039868023632579i, "z(inf)"=0.06039868023632579-0.47333723920034887i, "z (pi/2)"=0.47333723920034887+0.05239868023632578i, "z center"=0.0040000000000000036-0.0040000000000000036i, "z(0)"=-0.05239868023632578+0.46533723920034886i, "radius"=0.47271371381905647}}, "timestamp(min)"=857.1333333328366, "timestamp"=timestamp(3493779249 s since 1904-01-01), "Magn Field(T)"=0.0}, {"temperature"=77.83, "lorentzian"={"Amplitude"=0.00032563005286835036, "omega(0)"=665.1126173659541, "Gamma"=0.03556002784230838, "phase"=3.399487769267025, "Q"=18703.939724552765, "Norm  Ampl"=0.016702920764940257, "z (inf)"=0.13979772782045274-0.4501767488197134i, "4corners"={"z (-pi/2)"=-0.4341767488197134-0.11579772782045272i, "z(inf)"=0.13979772782045274-0.4501767488197134i, "z (pi/2)"=0.47417674881971345+0.12379772782045273i, "z center"=0.020000000000000018+0.0040000000000000036i, "z(0)"=-0.09979772782045271+0.45817674881971343i, "radius"=0.4697105648794674}}, "timestamp(min)"=858.4500000029802, "timestamp"=timestamp(3493779328 s since 1904-01-01), "Magn Field(T)"=0.0}, {"temperature"=77.749, "lorentzian"={"Amplitude"=0.00031222883825772935, "omega(0)"=665.0915026087613, "Gamma"=0.03382459230741114, "phase"=3.3211169604840762, "Q"=19662.95695641057, "Norm  Ampl"=0.014852241830341355, "z (inf)"=0.034405653249216225-0.4360391366695436i, "4corners"={"z (-pi/2)"=-0.47603913666954356-0.08240565324921621i, "z(inf)"=0.034405653249216225-0.4360391366695436i, "z (pi/2)"=0.3880391366695436+0.0744056532492162i, "z center"=-0.043999999999999984-0.0040000000000000036i, "z(0)"=-0.12240565324921619+0.4280391366695436i, "radius"=0.43909595998551487}}, "timestamp(min)"=859.7666666656733, "timestamp"=timestamp(3493779407 s since 1904-01-01), "Magn Field(T)"=0.0}, {"temperature"=77.673, "lorentzian"={"Amplitude"=0.0002968693327402179, "omega(0)"=665.0706732652532, "Gamma"=0.03218971740677334, "phase"=3.260073952151184, "Q"=20660.966508681107, "Norm  Ampl"=0.015285240009963012, "z (inf)"=0.04412913337028084-0.4755195090008862i, "4corners"={"z (-pi/2)"=-0.4835195090008862-0.060129133370280856i, "z(inf)"=0.04412913337028084-0.4755195090008862i, "z (pi/2)"=0.4595195090008862+0.05212913337028085i, "z center"=-0.01200000000000001-0.0040000000000000036i, "z(0)"=-0.06812913337028087+0.4675195090008862i, "radius"=0.47484853056668036}}, 
